vi "XML_Data_Set.vi"(10 "User Input":string[](array[string]), 11 "DOM document in":refnum<k20>) -> (2 "XML Output":string, 3 "OwnerDocument":refnum<k20>)   [LabVIEW 2009]
uses:
  Program Files/National Instruments/LabVIEW 2009/resource/objmgr/DOMUserDefRef.rc
  <vilib>/xml/NI_XML.lvlib
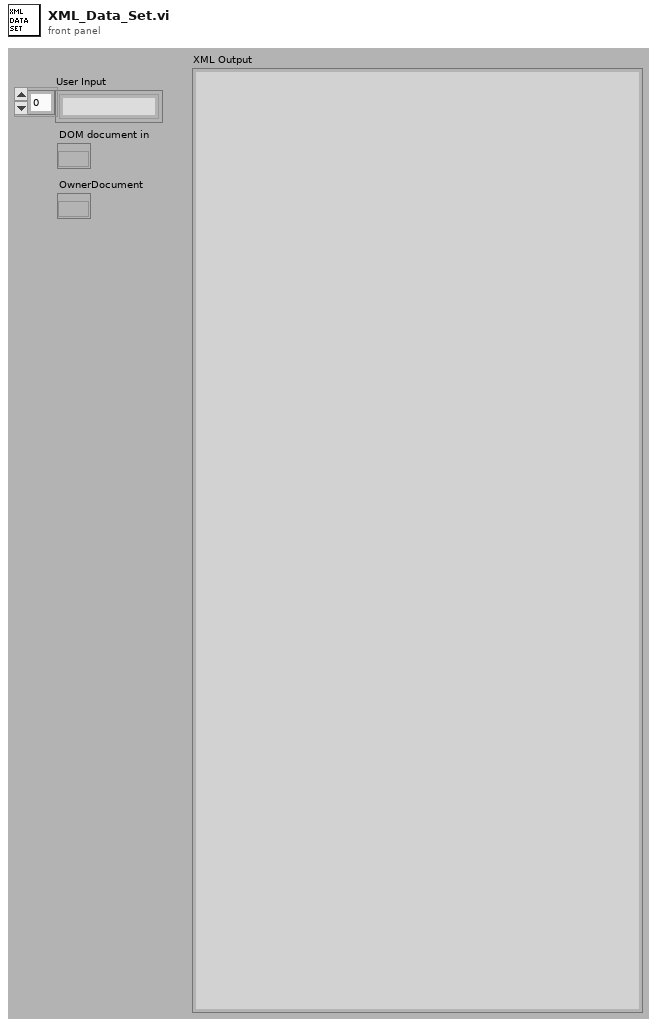
[diagram p1: front panel]
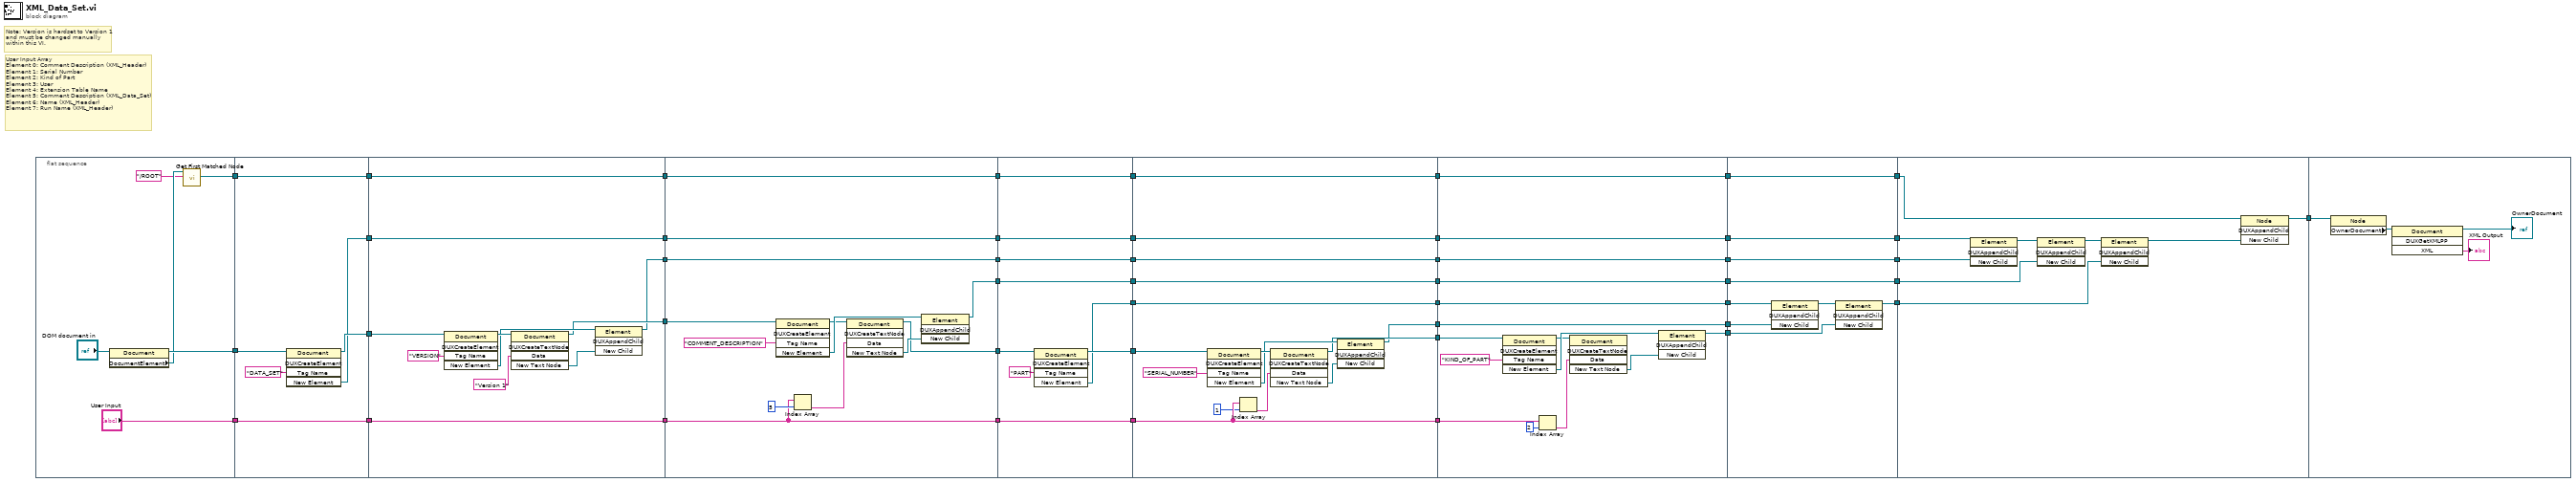
[diagram p0: block diagram]
diagram:
  # "User Input Array\nElement 0: Comment Description (XML_Header)\nElement 1: Serial Number\nElement 2: Kind of Part\nElement 3: User\nElement 4: Extension Table Name\nElement 5: Comment Description (XML_Data_Set)\nElement 6: Name (XML_Header)\nElement 7: Run Name (XML_Header)"
  # "Note: Version is hardset to Version 1\nand must be changed manually \nwithin this VI."
  n1 = flat-sequence {
    tunnel: [w51] -> w46
    tunnel: [w48] -> w35
    tunnel: ["User Input"] -> w14
    tunnel: w46 -> [w57]
    tunnel: [w56] -> w45
    tunnel: [w55] -> w36
    tunnel: w35 -> [w55]
    tunnel: [w54] -> w20
    tunnel: [w53] -> w15
    tunnel: w14 -> [w53]
    tunnel: w45 -> [w67]
    tunnel: [w63] -> w44
    tunnel: [w62] -> w37
    tunnel: w36 -> [w62]
    tunnel: [w61] -> w25
    tunnel: [w60] -> w24
    tunnel: w20 -> [w60]
    tunnel: [w59] -> w16
    tunnel: w15 -> [w59]
    tunnel: w44 -> [w78]
    tunnel: [w77] -> w43
    tunnel: [w76] -> w38
    tunnel: w37 -> [w76]
    tunnel: [w75] -> w29
    tunnel: [w74] -> w26
    tunnel: w25 -> [w74]
    tunnel: w24 -> [w73]
    tunnel: [w73] -> w23
    tunnel: [w71] -> w17
    tunnel: w16 -> [w71]
    tunnel: w43 -> [w90]
    tunnel: [w89] -> w42
    tunnel: [w88] -> w39
    tunnel: w38 -> [w88]
    tunnel: [w87] -> w32
    tunnel: [w86] -> w30
    tunnel: w29 -> [w86]
    tunnel: [w85] -> w27
    tunnel: w26 -> [w85]
    tunnel: w23 -> [w84]
    tunnel: [w84] -> w22
    tunnel: [w83] -> w18
    tunnel: w17 -> [w83]
    tunnel: w42 -> [w102]
    tunnel: [w101] -> w41
    tunnel: [w100] -> w40
    tunnel: w39 -> [w100]
    tunnel: [w99] -> w34
    tunnel: [w98] -> w33
    tunnel: w32 -> [w98]
    tunnel: [w97] -> w31
    tunnel: w30 -> [w97]
    tunnel: [w96] -> w28
    tunnel: w27 -> [w96]
    tunnel: w22 -> [w95]
    tunnel: [w95] -> w21
    tunnel: [w94] -> w19
    tunnel: w18 -> [w94]
    tunnel: w41 -> [w118]
    tunnel: [w116] -> w12
    tunnel: w40 -> [w116]
    tunnel: [w115] -> w10
    tunnel: [w114] -> w9
    tunnel: w34 -> [w114]
    tunnel: [w113] -> w8
    tunnel: w33 -> [w113]
    tunnel: [w112] -> w7
    tunnel: w31 -> [w112]
    tunnel: [w111] -> w5
    tunnel: w28 -> [w111]
    tunnel: w21 -> [w110]
    tunnel: [w110] -> w3
    tunnel: w19 -> [w107]
    tunnel: w12 -> [w130]
    tunnel: [w130] -> w11
    tunnel: w10 -> [w124]
    tunnel: w9 -> [w123]
    tunnel: w8 -> [w126]
    tunnel: w7 -> [w129]
    tunnel: [w129] -> w6
    tunnel: w5 -> [w128]
    tunnel: [w128] -> w4
    tunnel: w3 -> [w127]
    tunnel: [w127] -> w2
    tunnel: [w122] -> w1
    tunnel: w11 -> [w131]
    tunnel: w6 -> [w134]
    tunnel: w4 -> [w136]
    tunnel: w2 -> [w137]
    tunnel: [w138] -> w13
    tunnel: w1 -> [w133]
    tunnel: w13 -> [w140]
    frame #0 {
      n2 = property class="Document"(reference="DOM document in") -> (reference out=w51:refnum<k20>, "DocumentElement"=w50:refnum<k20>)  [unwired: 1 in, 1 out]
      n3 = call <vilib>:"Get First Matched Node.vi"("XPath expression"="/ROOT", "node in"=w50) -> ("node result"=w48:refnum<k20>)  [unwired: 7 in, 2 out]
    }
    frame #1 {
      n4 = invoke class="Document" method="DUXCreateElement"(reference=w57, "Tag Name"="DATA_SET") -> (reference out=w56:refnum<k20>, "New Element"=w54:refnum<k20>)  [unwired: 3 in, 3 out]
    }
    frame #2 {
      n5 = invoke class="Document" method="DUXCreateElement"(reference=w67, "Tag Name"="VERSION") -> (reference out=w66:refnum<k20>, "New Element"=w64:refnum<k20>)  [unwired: 3 in, 3 out]
      n6 = invoke class="Document" method="DUXCreateTextNode"(reference=w66, "Data"="Version 1") -> (reference out=w63:refnum<k20>, "New Text Node"=w65:refnum<k20>)  [unwired: 3 in, 3 out]
      n7 = invoke class="Element" method="DUXAppendChild"(reference=w64, "New Child"=w65) -> (reference out=w61:refnum<k20>)  [unwired: 2 in, 3 out]
    }
    frame #3 {
      n8 = invoke class="Document" method="DUXCreateElement"(reference=w78, "Tag Name"="COMMENT_DESCRIPTION") -> (reference out=w80:refnum<k20>, "New Element"=w82:refnum<k20>)  [unwired: 3 in, 3 out]
      n9 = Index Array(array=w71, index=5) -> (element=w70:string)
      n10 = invoke class="Document" method="DUXCreateTextNode"(reference=w80, "Data"=w70) -> (reference out=w77:refnum<k20>, "New Text Node"=w81:refnum<k20>)  [unwired: 3 in, 3 out]
      n11 = invoke class="Element" method="DUXAppendChild"(reference=w82, "New Child"=w81) -> (reference out=w75:refnum<k20>)  [unwired: 2 in, 3 out]
    }
    frame #4 {
      n12 = invoke class="Document" method="DUXCreateElement"(reference=w90, "Tag Name"="PART") -> (reference out=w89:refnum<k20>, "New Element"=w87:refnum<k20>)  [unwired: 3 in, 3 out]
    }
    frame #5 {
      n13 = invoke class="Document" method="DUXCreateElement"(reference=w102, "Tag Name"="SERIAL_NUMBER") -> (reference out=w106:refnum<k20>, "New Element"=w104:refnum<k20>)  [unwired: 3 in, 3 out]
      n14 = Index Array(array=w94, index=1) -> (element=w92:string)
      n15 = invoke class="Document" method="DUXCreateTextNode"(reference=w106, "Data"=w92) -> (reference out=w101:refnum<k20>, "New Text Node"=w103:refnum<k20>)  [unwired: 3 in, 3 out]
      n16 = invoke class="Element" method="DUXAppendChild"(reference=w104, "New Child"=w103) -> (reference out=w99:refnum<k20>)  [unwired: 2 in, 3 out]
    }
    frame #6 {
      n17 = invoke class="Document" method="DUXCreateElement"(reference=w118, "Tag Name"="KIND_OF_PART") -> (reference out=w119:refnum<k20>, "New Element"=w120:refnum<k20>)  [unwired: 3 in, 3 out]
      n18 = Index Array(array=w107, index=2) -> (element=w108:string)
      n19 = invoke class="Document" method="DUXCreateTextNode"(reference=w119, "Data"=w108) -> ("New Text Node"=w117:refnum<k20>)  [unwired: 3 in, 4 out]
      n20 = invoke class="Element" method="DUXAppendChild"(reference=w120, "New Child"=w117) -> (reference out=w115:refnum<k20>)  [unwired: 2 in, 3 out]
    }
    frame #7 {
      n21 = invoke class="Element" method="DUXAppendChild"(reference=w126, "New Child"=w123) -> (reference out=w125:refnum<k20>)  [unwired: 2 in, 3 out]
      n22 = invoke class="Element" method="DUXAppendChild"(reference=w125, "New Child"=w124) -> (reference out=w122:refnum<k20>)  [unwired: 2 in, 3 out]
    }
    frame #8 {
      n23 = invoke class="Element" method="DUXAppendChild"(reference=w137, "New Child"=w136) -> (reference out=w135:refnum<k20>)  [unwired: 2 in, 3 out]
      n24 = invoke class="Element" method="DUXAppendChild"(reference=w135, "New Child"=w134) -> (reference out=w132:refnum<k20>)  [unwired: 2 in, 3 out]
      n25 = invoke class="Element" method="DUXAppendChild"(reference=w132, "New Child"=w133) -> (reference out=w139:refnum<k20>)  [unwired: 2 in, 3 out]
      n26 = invoke class="Node" method="DUXAppendChild"(reference=w131, "New Child"=w139) -> (reference out=w138:refnum<k20>)  [unwired: 2 in, 3 out]
    }
    frame #9 {
      n27 = property class="Node"(reference=w140) -> ("OwnerDocument"=w141:refnum<k20>)  [unwired: 1 in, 2 out]
      n28 = invoke class="Document" method="DUXGetXMLPP"(reference=w141) -> (reference out=→"OwnerDocument":refnum<k20>, "XML"=→"XML Output":string)  [unwired: 3 in, 2 out]
    }
  }
